vi "rttrace.vi"() -> ()   [LabVIEW 2013]
uses:
  errors/severity.ctl
  errors/exception.lvlib
  <vilib>/platform/TimedLoop/XDataNode/XDataNode.xnode
  <vilib>/Platform/TimedLoop/XDataNode/nitl_modes.ctl
  <vilib>/Platform/TimedLoop/XDataNode/XDNodeRunTimeDep.lvlib
  <vilib>/Platform/TimedLoop/XDataNode/wakeup.ctl
  <vilib>/Platform/TimedLoop/XDataNode/timing_clust.ctl
  errors/exception.ctl
  errors/context.ctl
panel:
  out "String":string
  out "properties":variant
  in  "code":i32
  out "exception out 2":T1 {"code" format="%.0x"}
  out "error out":errorcluster
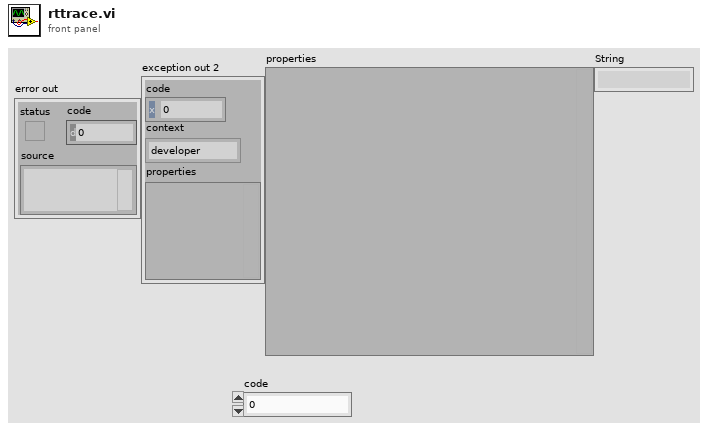
[diagram p1: front panel]
types:
  T1 = typedef "exception.lvlib/exception.ctl" = cluster{"code":i32, "context":T2, "properties":variant}
  T2 = typedef "exception.lvlib/context.ctl" = enum16{"developer", "user interface", "standard", "limited", "deterministic"}
  T3 = typedef "exception.lvlib/severity.ctl" = enum8{"unspecified", "operation failed", "data corruption", "system corruption", "critical unknown state"}
  T4 = typedef "XDNodeRunTimeDep.lvlib/timing_clust.ctl" = cluster{"Expected End [f-1]":u64, "Actual End [f-1]":u64, "Finished Late? [f-1]":bool, "Expected End [i-1]":u64, "Actual End [i-1]":u64, "Finished Late? [i-1]":bool, "Expected Start [i]":u64, "Actual Start [i]":u64, "Expected Start [f]":u64, "Actual Start [f]":u64, "Source Name":string, "Structure Name":string, "Period":i64, "Deadline":i64, "Offset":i64, "Start":i64, "Priority":i32, "Timeout":i32, "Mode":T5, "Wakeup Reason":T6, "Error":errorcluster, "Source Type":string, "Secondary Source Type":string, "Global End Time":u64, "Global Start Time":u64, "Frame Duration":u64, "Iteration Duration":u64, "Assigned CPU":i32, "I/O Scan Engine Mode":u32}
  T5 = typedef "XDNodeRunTimeDep.lvlib/nitl_modes.ctl" = enum32{"No Change", "Process missed periods, maintain original phase", "Discard missed periods, maintain original phase", "Process missed periods, ignore original phase", "Discard missed periods, ignore original phase"}
  T6 = typedef "XDNodeRunTimeDep.lvlib/wakeup.ctl" = enum32{"Normal", "Aborted", "Asynchronous wakeup", "Timing source error", "Timed loop error", "Timeout"}
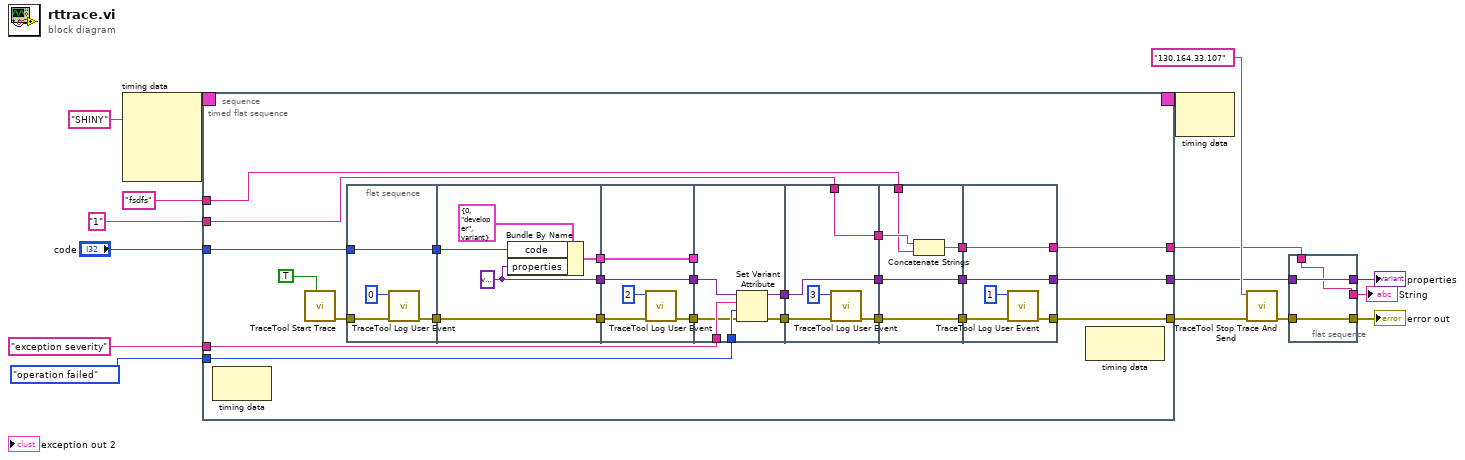
[diagram p0: block diagram]
diagram:
  n1 = node-c288("SHINY" ("Structure Name")) -> (w16:T4)  [unwired: 3 in]
  n2 = timed-sequence {
    timing: w16 -> [_]
    timing-out: [_] -> w15
    tunnel: [w24] -> w10
    tunnel: [w23] -> w9
    tunnel: "code" -> [w22]
    tunnel: severity."operation failed" ("severity 2") -> [w21]
    tunnel: "exception severity" -> [w20]
    tunnel: "1" -> [w19]
    tunnel: "fsdfs" -> [w18]
    tunnel: [w17] -> w2
    n3 = timed-flat-sequence {
      tunnel: [w44] -> w24
      tunnel: [w43] -> w23
      tunnel: w22 -> [w34]
      tunnel: w21 -> [w33]
      tunnel: w20 -> [w32]
      tunnel: w19 -> [w28]
      tunnel: w18 -> [w27]
      tunnel: [w26] -> w17
      n4 = node-c288() -> ()  [unwired: 1 in, 1 out]
      n5 = call <vilib>:"TraceTool Start Trace.vi"("Detailed Tracing? (F)"=TRUE) -> ("error out"=w46:errorcluster)  [unwired: 9 in, 1 out]
      n6 = flat-sequence {
        tunnel: w46 -> [w54]
        tunnel: [w53] -> w50
        tunnel: [w51] -> w35
        tunnel: w34 -> [w51]
        tunnel: w50 -> [w59]
        tunnel: [w59] -> w49
        tunnel: [w57] -> w40
        tunnel: w35 -> [w56]
        tunnel: [w55] -> w30
        tunnel: w49 -> [w64]
        tunnel: [w63] -> w48
        tunnel: [w61] -> w41
        tunnel: w40 -> [w61]
        tunnel: [w60] -> w31
        tunnel: w30 -> [w60]
        tunnel: w48 -> [w66]
        tunnel: [w65] -> w47
        tunnel: [w67] -> w42
        tunnel: w41 -> [_]
        tunnel: w33 -> [w70]
        tunnel: w32 -> [w69]
        tunnel: w31 -> [w68]
        tunnel: w47 -> [w75]
        tunnel: [w74] -> w39
        tunnel: [w72] -> w37
        tunnel: w42 -> [w72]
        tunnel: [w71] -> w29
        tunnel: w28 -> [w71]
        tunnel: w39 -> [w80]
        tunnel: [w80] -> w38
        tunnel: w37 -> [w79]
        tunnel: [w79] -> w36
        tunnel: w29 -> [w78]
        tunnel: w27 -> [w77]
        tunnel: [w76] -> w25
        tunnel: [w84] -> w44
        tunnel: w38 -> [w85]
        tunnel: [w82] -> w43
        tunnel: w36 -> [w82]
        tunnel: [w81] -> w26
        tunnel: w25 -> [w81]
        frame #0 {
          n7 = call <vilib>:"TraceTool Log User Event.vi"("error in (no error)"=w54, "Event ID (0-255)"=u32 0) -> ("error out"=w53:errorcluster)  [unwired: 9 in]
        }
        frame #1 {
          w55 = variant ("properties")
          n8 = Bundle By Name(cluster=T1 {"code"=0, "context"=enum."developer", "properties"=variant} ("exception"), "code"=w56, "properties"=w55) -> (w57:T1)
        }
        frame #2 {
          n9 = call <vilib>:"TraceTool Log User Event.vi"("error in (no error)"=w64, "Event ID (0-255)"=u32 2) -> ("error out"=w63:errorcluster)  [unwired: 9 in]
        }
        frame #3 {
          n10 = Set Variant Attribute(Variant=w68, name=w69, value=w70, error in=w66) -> (Variant out=w67:variant, error out=w65:errorcluster)  [unwired: 1 out]
        }
        frame #4 {
          n11 = call <vilib>:"TraceTool Log User Event.vi"("error in (no error)"=w75, "Event ID (0-255)"=u32 3) -> ("error out"=w74:errorcluster)  [unwired: 9 in]
        }
        frame #5 {
          n12 = Concatenate Strings(w78, w77) -> (w76:string)
        }
        frame #6 {
          n13 = call <vilib>:"TraceTool Log User Event.vi"("error in (no error)"=w85, "Event ID (0-255)"=u32 1) -> ("error out"=w84:errorcluster)  [unwired: 9 in]
        }
      }
      n14 = node-c288() -> ()  [unwired: 1 in, 1 out]
    }
  }
  n15 = node-c288(w15) -> ()  [unwired: 1 out]
  n16 = call <vilib>:"TraceTool Stop Trace And Send.vi"("error in (no error)"=w10, "Trace Host Network Address"="130.164.33.107") -> ("error out"=w12:errorcluster)  [unwired: 9 in]
  n17 = flat-sequence {
    tunnel: w12 -> [w90]
    tunnel: [w90] -> w13
    tunnel: [w89] -> w6
    tunnel: w9 -> [w89]
    tunnel: [w88] -> w1
    tunnel: w2 -> [w88]
    frame #0 {
    }
  }
  "error out" <- w13
  "properties" <- w6
  "String" <- w1
